vi "hist_icp.vi"(11 "sensor_obs":dbl[](array[numeric])) -> (0 "Histogram Graph":T1(graph), 3 "out":dbl[](array[numeric]))   [LabVIEW 2012]
uses:
  <vilib>/Analysis/NI_AALBase.lvlib
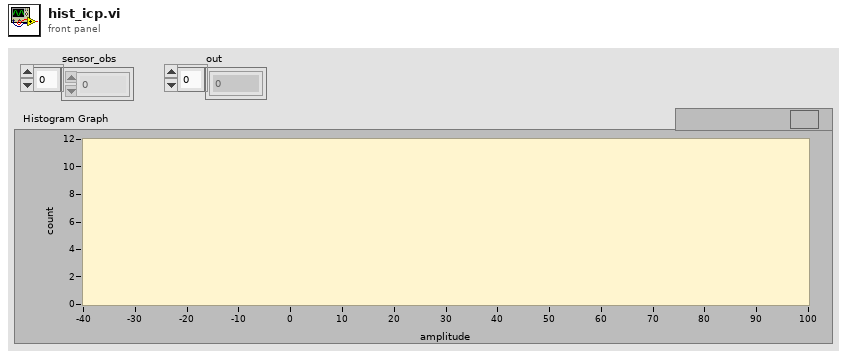
[diagram p1: front panel]
types:
  T1 = cluster{"X Values":dbl[], "Histogram: h(x)":i32[]}
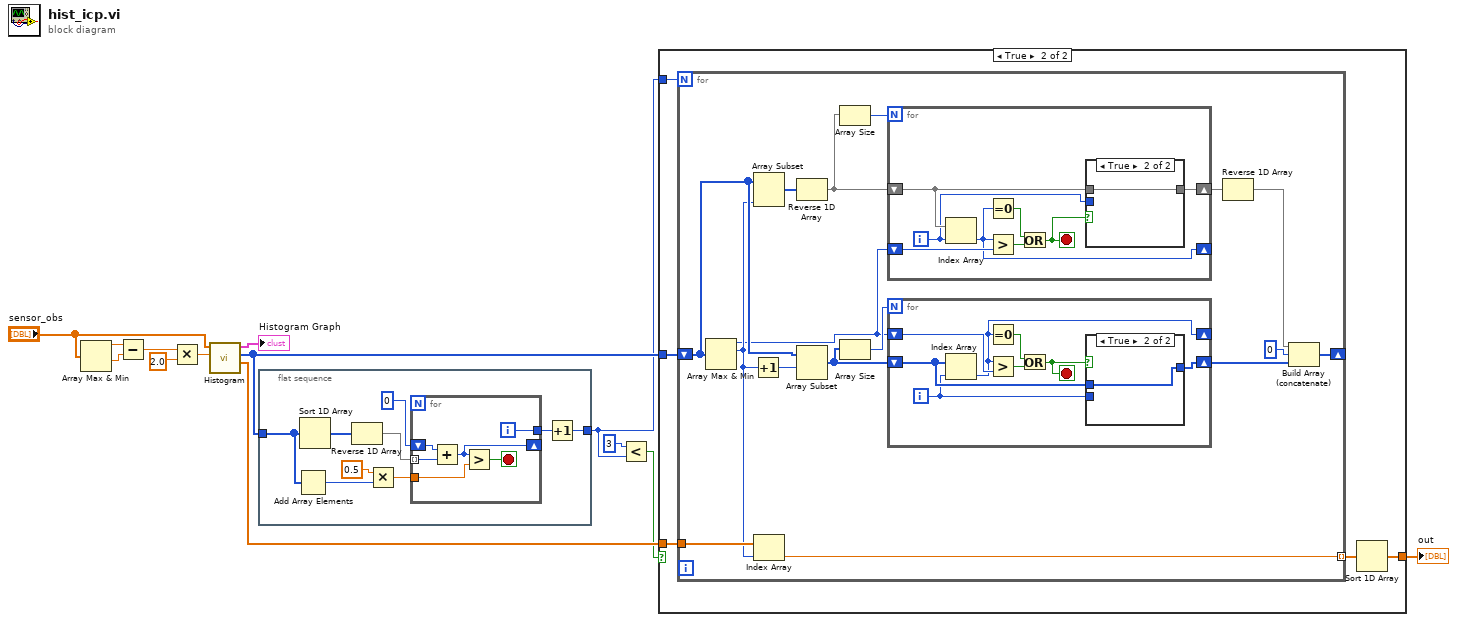
[diagram p0: block diagram]
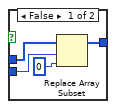
[diagram p3: hidden frame]
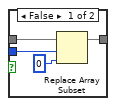
[diagram p4: hidden frame]
diagram:
  n1 = Array Max & Min(array="sensor_obs") -> (max value=w5:dbl, min value=w6:dbl)  [unwired: 2 out]
  n2 = Subtract(x=w5, y=w6) -> (x-y=w9:dbl)
  n3 = Multiply(x=w9, y=2.0) -> (x*y=w11:dbl)
  n4 = call <vilib>:"Histogram.vi"("intervals"=w11, "X"="sensor_obs") -> ("X Values"=w8:dbl[], "Histogram: h(x)"=w13:i32[], "Histogram Graph"=→"Histogram Graph":T1)  [unwired: 6 in, 1 out]
  n5 = flat-sequence {
    tunnel: w13 -> [w22]
    tunnel: [w14] -> w3
    frame #0 {
      n6 = Add Array Elements(numeric array=w22) -> (sum=w20:i32)
      n7 = Sort 1D Array(array=w22) -> (sorted array=w21:i32[])
      n8 = Reverse 1D Array(array=w21) -> (reversed array=w18:i32[])
      n9 = Multiply(x=0.5, y=w20) -> (x*y=w17:dbl)
      n10 = for {
        tunnel: w18 -> [w27] mode=indexing
        tunnel: w17 -> [w25]
        shift-right: [w26] -> _
        shift-left: 0 -> [w28]
        tunnel: [w23] -> w15
        i -> [w23]
        stop <- w24 stop-if-true
        n11 = Add(x=w28, y=w27) -> (x+y=w26:i32)
        n12 = Greater?(x=w26, y=w25) -> (0:w24:bool)
      }
      n13 = Increment(x=w15) -> (x+1=w14:i32)
    }
  }
  n14 = Less?(x=3, y=w3) -> (x < y?=w1:bool)
  n15 = case shown="True" w1 {
    tunnel: w13 -> [_ w33]
    tunnel: [_ w32] -> w12
    tunnel: w8 -> [_ w30]
    tunnel: w3 -> [_ w29]
    frame False {
    }
    frame True {
      n16 = for {
        N: w29 -> [_]
        shift-right: [w38] -> _
        shift-left: w33 -> [w49]
        tunnel: w30 -> [w37]
        tunnel: [w35] -> w31 mode=indexing
        n17 = Array Max & Min(array=w49) -> (max value=w34:i32, max index (indices)=w36:i32)  [unwired: 2 out]
        n18 = Increment(x=w36) -> (x+1=w47:i32)
        n19 = Array Subset(array=w49, length=w36) -> (w48:i32[])  [unwired: 1 in]
        n20 = Index Array(array=w37, index=w36) -> (element=w35:dbl)
        n21 = Reverse 1D Array(array=w48) -> (reversed array=w46:i32[])
        n22 = Array Subset(array=w49, index=w47) -> (w42:i32[])  [unwired: 1 in]
        n23 = Array Size(array=w46) -> (size(s)=w45:i32)
        n24 = Array Size(array=w42) -> (size(s)=w43:i32)
        n25 = for {
          N: w45 -> [_]
          shift-right: [w66] -> _
          shift-left: w34 -> [w70]
          shift-right: [w67] -> w44
          shift-left: w46 -> [w69]
          i -> [w68]
          stop <- w63 stop-if-true
          n26 = Index Array(array=w69, index=w68) -> (element=w66:i32)
          n27 = Equal To 0?(x=w66) -> (x = 0?=w65:bool)
          n28 = Greater?(x=w66, y=w70) -> (0:w64:bool)
          n29 = Or(x=w65, y=w64) -> (x .or. y?=w63:bool)
          n30 = case shown="True" w63 {
            tunnel: w69 -> [w74 w75]
            tunnel: w68 -> [w73 _]
            tunnel: [w72 w75] -> w67
            frame False {
              n31 = Replace Array Subset(array=w74, new element=0 ("new element/subarray"), index=w73) -> (w72:i32[])
            }
            frame True {
            }
          }
        }
        n32 = for {
          N: w43 -> [_]
          shift-right: [w53] -> _
          shift-left: w34 -> [w57]
          shift-right: [w54] -> w40
          shift-left: w42 -> [w56]
          i -> [w55]
          stop <- w50 stop-if-true
          n33 = Index Array(array=w56, index=w55) -> (element=w53:i32)
          n34 = Equal To 0?(x=w53) -> (x = 0?=w52:bool)
          n35 = Greater?(x=w53, y=w57) -> (0:w51:bool)
          n36 = Or(x=w52, y=w51) -> (x .or. y?=w50:bool)
          n37 = case shown="True" w50 {
            tunnel: w56 -> [w61 w62]
            tunnel: w55 -> [w60 _]
            tunnel: [w59 w62] -> w54
            frame False {
              n38 = Replace Array Subset(array=w61, new element=0 ("new element/subarray"), index=w60) -> (w59:i32[])
            }
            frame True {
            }
          }
        }
        n39 = Reverse 1D Array(array=w44) -> (reversed array=w41:i32[])
        n40 = Build Array (concatenate)(w41, 0, w40) -> (w38:i32[])
      }
      n41 = Sort 1D Array(array=w31) -> (sorted array=w32:dbl[])
    }
  }
  "out" <- w12
